vi "Trav_single_profile.vi"(3 "Simulate/Run":T1, 5 "Traverse line":T2 {"Row Duration (mins)" format="%#.1f"; "Row No" min=0; "Trace Gas Concentration (%)" min=0.0 format="%#.2f"; "Emission Rate (l/min)" format="%#.2f"; "Tunnel Speed" format="%#.2f"; "Start X" format="%#.2f"; "Start Y" format="%#.2f"; "Start Z" format="%#.2f"; "End X" format="%#.2f"; "End Y" format="%#.2f"; "End Z" format="%#.2f"; "Averaging time (min)" min=0.0 format="%#.2f"}) -> (0 "Error Messages":string, 1 "Status":T5, 2 "Traverse line Out":T2 {"Row Duration (mins)" format="%#.1f"; "Row No" min=0; "Trace Gas Concentration (%)" min=0.0 format="%#.2f"; "Emission Rate (l/min)" format="%#.2f"; "Tunnel Speed" format="%#.2f"; "Start X" format="%#.2f"; "Start Y" format="%#.2f"; "Start Z" format="%#.2f"; "End X" format="%#.2f"; "End Y" format="%#.2f"; "End Z" format="%#.2f"; "Averaging time (min)" min=0.0 format="%#.2f"})   [LabVIEW 2011]
uses:
  Gen Trav/Multi_Run_Status.ctl
  Gen Trav/Traverse_cluster.ctl
  Gen Trav/Spacing.ctl
  Controls/Multi_run_mode.ctl
  Controls/User_Specific_mode.ctl
  Controls/Save_Data.ctl
  Controls/Setup.ctl
  ADAM Client/Sub VIs/ADAM Controls/Traverse_Level_State.ctl
  Controls/Overhead.ctl
  Globals/Trav_pos_global.vi
  Globals/Meas_global.vi
panel:
  out "Pause message":string
  in  "Pause":bool
  out "Current position":dbl[](array[numeric]) format="%.2f"
  in  "Stop":bool
  in  "Array of Positions":dbl[][](array[numeric]) format="%.2f"
  out "Abcissa copy":string="Y (mm)"
  out "Abcissa":string="Y (mm)"
  in  "ChannelsToPlot":i32[](listbox)=[1]
  out "Started Profile at:":string="16/9/98 12:33"
  out "Currently on point":i32=9
  out "Means":cluster{dbl[], dbl[]}[](graph)
  out "Turbulence%":cluster{dbl[], dbl[]}[](graph)
  # "X           Y            Z"
  # "Start"
  # "End"
  # "X           Y            Z"
  # "Start"
  # "End"
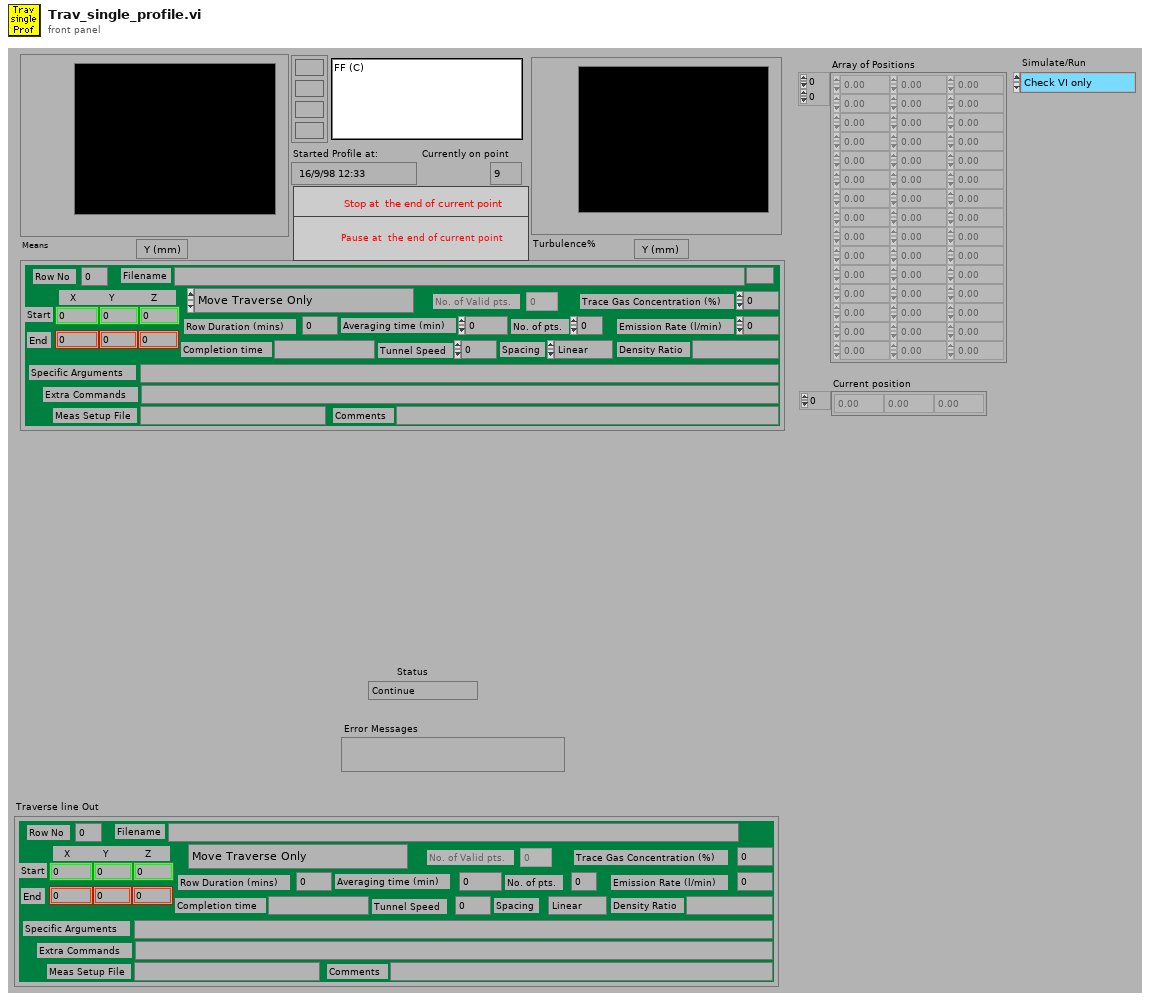
[diagram p1: front panel]
types:
  T1 = typedef "User_Specific_mode.ctl" = enum16{"Check VI only", "Run VI"}
  T2 = typedef "Traverse_cluster.ctl" = cluster{"Start X":dbl, "Start Y":dbl, "Start Z":dbl, "End X":dbl, "End Y":dbl, "End Z":dbl, "No. of pts.":i32, "Spacing":T3, "Filename":path, "Tunnel Speed":dbl, "Averaging time (min)":dbl, "Extra Commands":string, "Specific Arguments":string, "Emission Rate (l/min)":dbl, "Trace Gas Concentration (%)":dbl, "Density Ratio":string, "Comments":string, "Row No":i32, "Row Type Selector":T4, "Completion time":string, "Row Duration (mins)":dbl, "No. of Valid pts.":i32, "Meas Setup File":string}
  T3 = typedef "Spacing.ctl" = enum16{"Linear", "Log", "Gauss", "Specified", "N/A"}
  T4 = typedef "Multi_run_mode.ctl" = enum16{"Move Traverse Only", "Set Tunnel Speed Only", "Set Source Only", "Set Measurement Conditions", "Single Measurement", "Vertical Profile", "Lateral Profile", "Longitudinal Profile", "Explore Volume", "Multi-Axis Profile", "Auto Calibrate", "Meas Fast FID Bkgnd", "Check Beam Power", "Scanning Valve Measurement", "Run VI Named:", "Set ADAM Ch", "Wait (minutes)", "Send Message", "Synchronize With:", "Fall Back to this Row", "Turn Off Row Repeating", "Blank Row", "Traverse 3D Volume"}
  T5 = typedef "Multi_Run_Status.ctl" = enum16{"Continue", "Jump to Next Point", "Jump to Next Row", "Jump To Fall Back", "Terminate Run"}
  T6 = typedef "Save_Data.ctl" = enum16{"Save No Data", "Save Data"}
  T7 = typedef "Setup.ctl" = enum16{"Run Program", "Show Setup", "Save Current Setup", "Setup Front Panel"}
  T8 = typedef "Traverse_Level_State.ctl" = enum16{"Running", "Complete"}
  T9 = typedef "Overhead.ctl" = enum16{"Update total times", "Read Current Overhead", "Re Scale totals to 3 hrs", "Initialise totals to 3hr"}
  T10 = typedef "Status_Cluster.ctl" = cluster{"Status":T5, "Error Type":string, "Error Description":string}
  T11 = typedef "Analysis_info_cluster.ctl" = cluster{"Colour":u32, "Inst type":T12, "Inst name":string, "Symbol":string, "Code name":string, "Extra Info":string, "Inst Array":T13, "Extra Titles":string[], "Extra Values":string[], "Eng Values":dbl[], "Time (ms)":dbl[], "Voltage":dbl[], "U":dbl, "u^2":dbl, "u^3":dbl, "u^4":dbl, "Skew_u":dbl, "Kurt_u":dbl, "Sd Error in Mean":dbl, "% u'/U":dbl, "X":dbl, "Y":dbl, "Z":dbl, "Spectra":T14, "Autocorrelation":T14, "Timescale integral to 25%":dbl, "Sd Error in Variance":dbl, "Calib File":path, "Calib Constants":dbl[], "Histogram":T14, "Output Position":bool, "Full Stats":bool, "Weighting":dbl[], "Av Sampling Rate":dbl, "Av No of Samples":dbl, "Total Meas Time (s)":dbl, "ADAM Ch Name":string}
  T12 = typedef "Inst_type.ctl" = enum16{"Propeller anemometer", "Raw voltage", "Pressure Transducer", "Pitot-static tube", "Preston tube", "Hot wire", "Cross wire 1", "Cross wire 2", "Generic Linear", "Generic Polynomial", "Generic BackPoly", "Fast FID", "Thermocouple", "Cold wire", "Pulsed Wire", "LDA Vel", "LDA Tran time", "LDA Arr time"}
  T13 = typedef "Instrument_Array.ctl" = enum16{"PWA", "LDA", "Analogue"}
  T14 = typedef "XY_Plot_Cluster.ctl" = cluster{"First Name":string, "Second Name":string, "X axis name":string, "Y axis name":string, "X array":dbl[], "Y array":dbl[]}
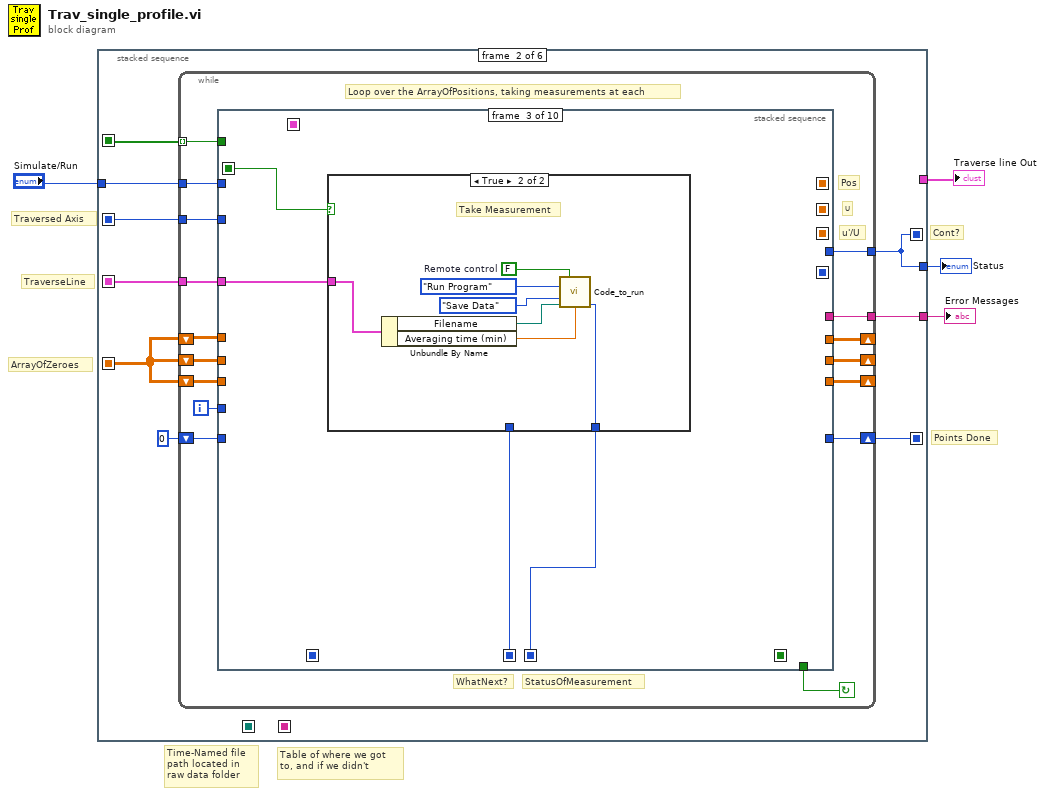
[diagram p0: block diagram]
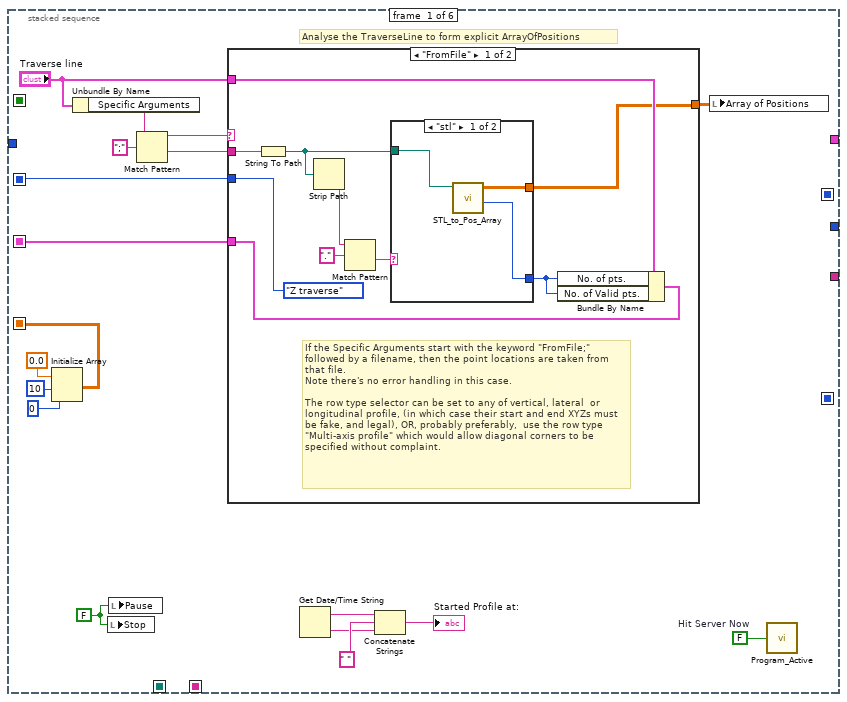
[diagram p2: hidden frame]
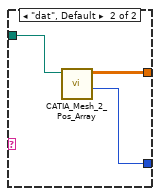
[diagram p3: hidden frame]
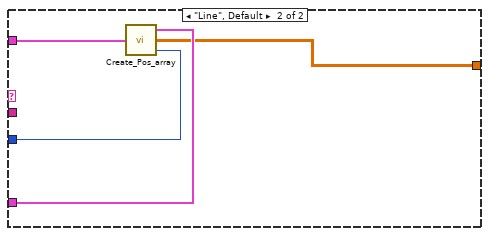
[diagram p4: hidden frame]
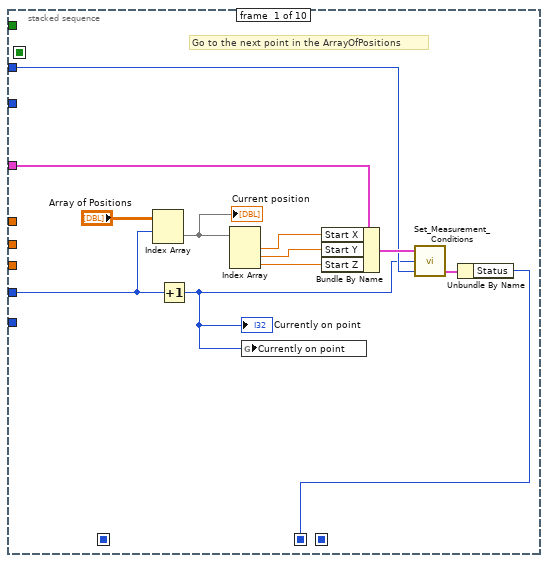
[diagram p5: hidden frame]
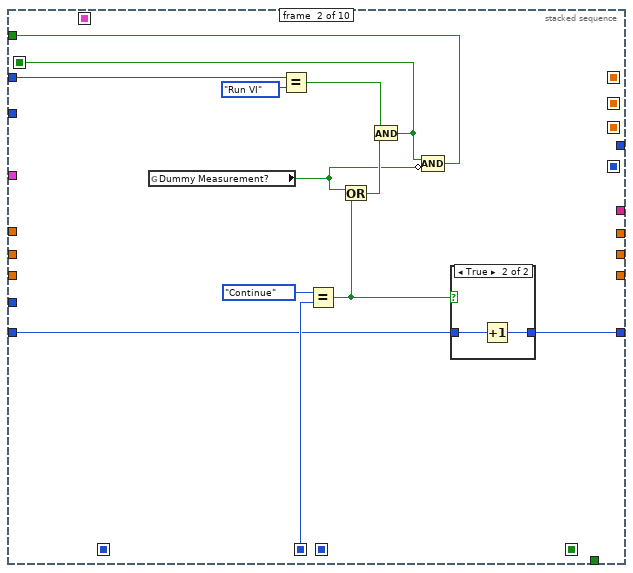
[diagram p6: hidden frame]
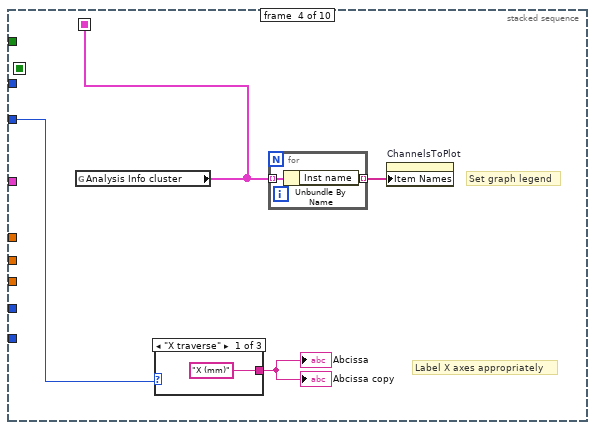
[diagram p9: hidden frame]
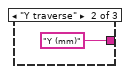
[diagram p10: hidden frame]
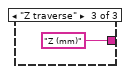
[diagram p11: hidden frame]
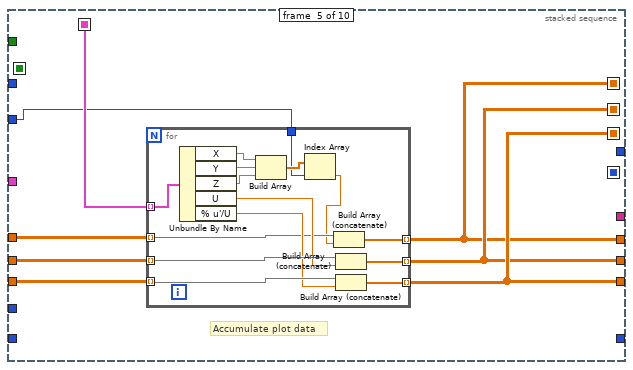
[diagram p12: hidden frame]
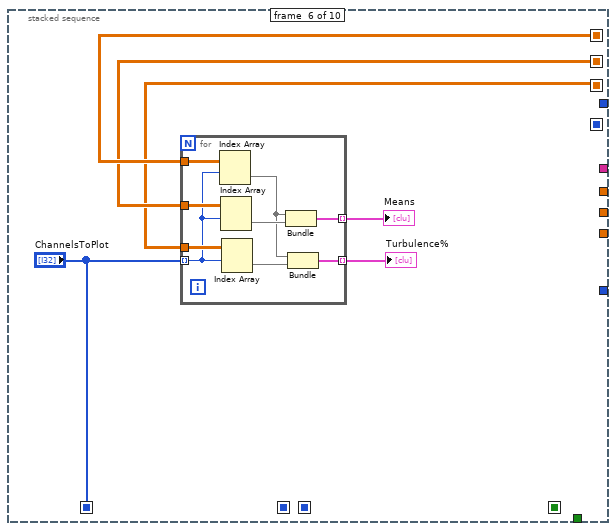
[diagram p13: hidden frame]
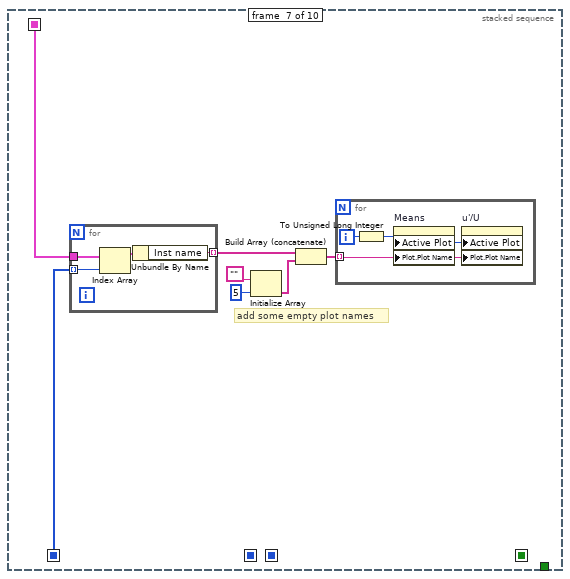
[diagram p14: hidden frame]
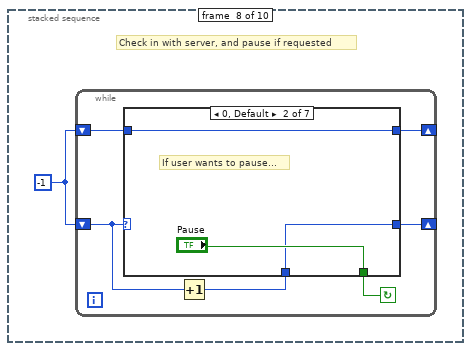
[diagram p15: hidden frame]
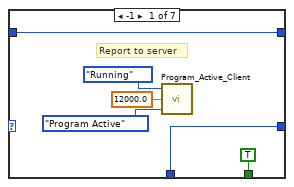
[diagram p16: hidden frame]
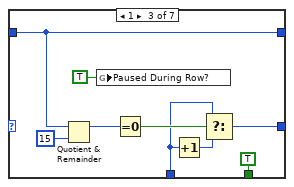
[diagram p17: hidden frame]
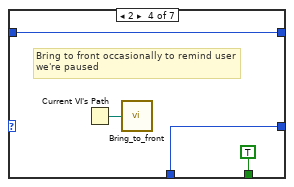
[diagram p18: hidden frame]
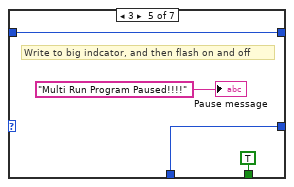
[diagram p19: hidden frame]
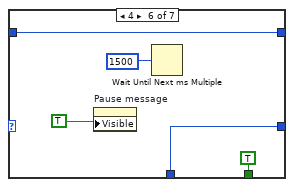
[diagram p20: hidden frame]
diagram:
  # "Table of where we got to, and if we didn't"
  # "Time-Named file path located in raw data folder"
  # "ArrayOfZeroes"
  # "TraverseLine"
  # "Traversed Axis"
  # "Points Done"
  # "Cont?"
  n1 = stacked-sequence {
    seq-local: [w15 _ _ _ _ _] -> [_ w50 _ _ _ _]
    seq-local: [w14 _ _ _ _ _] -> [_ w51 _ _ _ _]
    seq-local: [_ _ w272 _ _ _] -> [_ _ _ _ w296 _]
    seq-local: [_ _ _ w279 _ _] -> [_ _ _ _ w295 _]
    seq-local: [_ w49 _ _ _ _] -> [_ _ _ _ _ _]
    seq-local: [_ w47 _ _ _ _] -> [_ _ _ w276 w294 _]
    seq-local: [_ w45 _ _ _ _] -> [_ _ _ _ _ w301]
    seq-local: [w11 _ _ _ _ _] -> [_ w44 _ _ _ w303]
    tunnel: [_ w49 _ _ _ _] -> w2
    tunnel: [_ _ _ _ _ w313] -> w4
    tunnel: "Simulate/Run" -> [_ w48 _ _ _ w312]
    tunnel: [_ w43 _ _ _ _] -> w1
    frame #0 {
      w12 = FALSE ("stop")
      w13 = FALSE  # Hit Server Now
      # "Analyse the TraverseLine to form explicit ArrayOfPositions"
      n2 = Initialize Array(0.0, 10, 0) -> (w15:dbl[][])
      n3 = Unbundle By Name("Traverse line") -> ("Specific Arguments"=w8:string)
      n4 = local write "Stop"(w12) -> ()
      n5 = local write "Pause"(w12) -> ()
      n6 = Match Pattern(string=w8, regular expression=";") -> (before substring=w6:string, after substring=w5:string)  [unwired: 1 in, 2 out]
      n7 = case shown="\"FromFile\"" w6 {
        tunnel: [enum16{"X traverse", "Y traverse", "Z traverse"}."Z traverse" ("Axis Traversed") w42] -> w14
        tunnel: "Traverse line" -> [w26 w41]
        tunnel: [w25 w40] -> w11
        tunnel: [w23 w39] -> w10
        tunnel: w5 -> [w27 _]
        frame "FromFile" {
          # "If the Specific Arguments start with the keyword \"FromFile;\" followed by a filename, then the point locations are taken from that file.\nNote there's no error handling in this case.\n\nThe row type selector can be set to any of vertical, lateral  or longitudinal profile, (in which case their start and end XYZs must be fake, and legal), OR, probably preferably,  use the row type \"Multi-axis profile\" which would allow diagonal corners to be specified without complaint."
          n8 = String To Path(string=w27) -> (path=w29:path)
          n9 = Strip Path(path=w29) -> (name=w31:string)  [unwired: 1 out]
          n10 = Match Pattern(string=w31, regular expression=".") -> (after substring=w32:string)  [unwired: 1 in, 3 out]
          n11 = case shown="\"stl\"" w32 {
            tunnel: [w34 w38] -> w23
            tunnel: [w33 w37] -> w28
            tunnel: w29 -> [w35 w36]
            frame "stl" {
              n12 = call "STL_to_Pos_Array.vi"("STL file"=w35) -> ("Number of Points"=w33:i32, "Array of Positions"=w34:dbl[][])  [unwired: 9 in]
            }
            frame "dat", Default {
              n13 = call "CATIA_Mesh_2_Pos_Array.vi"("Catia Mesh File"=w36) -> ("Number of Points"=w37:i32, "Array of Positions"=w38:dbl[][])  [unwired: 9 in]
            }
          }
          n14 = Bundle By Name(cluster=w26, "No. of pts."=w28, "No. of Valid pts."=w28) -> (w25:T2)
        }
        frame "Line", Default {
          n15 = call "Create_Pos_array.vi"("Traverse line"=w41) -> ("Traverse line Out"=w40:T2, "Array of Positions"=w39:dbl[][], "Axis Traversed"=w42:enum16{"X traverse", "Y traverse", "Z traverse"})  [unwired: 5 in, 1 out]
        }
      }
      n16 = Get Date/Time String() -> (date string=w21:string, time string=w20:string)  [unwired: 3 out]
      n17 = Concatenate Strings(w21, " ", w20) -> (→"Started Profile at:":string)
      n18 = local write "Array of Positions"(w10) -> ()
      n19 = call "Program_Active.vi"("Hit Server Now"=w13) -> ()
    }
    frame #1 {
      n20 = while {
        shift-left: 0 -> [w54]
        shift-right: [w53] -> w45
        tunnel: [w55] -> w47 mode=indexing
        tunnel: w44 -> [w56]
        tunnel: w48 -> [w57]
        tunnel: [w58] -> w49
        shift-left: w50 -> [w61]
        shift-right: [w60] -> _
        tunnel: w51 -> [w62]
        shift-left: w50 -> [w64]
        shift-right: [w63] -> _
        shift-left: w50 -> [w66]
        shift-right: [w65] -> _
        tunnel: [w52] -> w43
        i -> [w67]
        stop <- w59 continue-if-true
        # "StatusOfMeasurement"
        # "WhatNext?"
        # "Loop over the ArrayOfPositions, taking measurements at each"
        # "Pos"
        # "U"
        # "u'/U"
        n21 = stacked-sequence {
          seq-local: [_ _ _ w107 _ _ _ _ _ _] -> [_ _ _ _ w121 _ w154 _ _ _]
          seq-local: [_ _ _ _ w117 _ _ _ _ _] -> [_ _ _ _ _ w144 _ _ _ _]
          seq-local: [_ _ _ _ w119 _ _ _ _ _] -> [_ _ _ _ _ w143 _ _ _ _]
          seq-local: [_ _ _ _ w120 _ _ _ _ _] -> [_ _ _ _ _ w142 _ _ _ _]
          seq-local: [_ _ _ _ _ "ChannelsToPlot" _ _ _ _] -> [_ _ _ _ _ _ w160 _ _ _]
          seq-local: [_ _ w98 _ _ _ _ _ _ _] -> [_ _ _ _ _ _ _ _ w221 _]
          seq-local: [w74 _ _ _ _ _ _ _ _ _] -> [_ w89 w96 _ _ _ _ _ _ _]
          seq-local: [_ w81 _ _ _ _ _ _ _ _] -> [_ _ w97 _ _ _ _ _ _ _]
          seq-local: [_ _ _ _ _ _ _ _ w216 _] -> [_ _ _ _ _ _ _ _ _ w228]
          seq-local: [_ _ _ _ _ _ _ _ w215 _] -> [_ _ _ _ _ _ _ _ _ w229]
          tunnel: w67 -> [w71 _ _ _ _ _ _ _ w224 w232]
          tunnel: w66 -> [_ _ _ _ w123 _ _ _ _ _]
          tunnel: [_ _ _ _ w119 _ _ _ _ _] -> w65
          tunnel: w64 -> [_ _ _ _ w122 _ _ _ _ _]
          tunnel: [_ _ _ _ w120 _ _ _ _ _] -> w63
          tunnel: w62 -> [_ _ _ w109 w116 _ _ _ _ _]
          tunnel: w61 -> [_ _ _ _ w118 _ _ _ _ _]
          tunnel: [_ _ _ _ w117 _ _ _ _ _] -> w60
          tunnel: [_ _ _ _ _ _ _ _ _ w228] -> w59
          tunnel: w56 -> [w78 _ w95 _ _ _ _ _ _ w233]
          tunnel: [_ _ _ _ _ _ _ _ _ w231] -> w58
          tunnel: w57 -> [w76 w91 _ _ _ _ _ _ _ w234]
          tunnel: [_ w82 _ _ _ _ _ _ _ _] -> w55
          tunnel: w54 -> [_ w86 _ _ _ _ _ _ _ _]
          tunnel: [_ w85 _ _ _ _ _ _ _ _] -> w53
          tunnel: [_ _ _ _ _ _ _ _ _ w230] -> w52
          frame #0 {
            # "Go to the next point in the ArrayOfPositions"
            n22 = Index Array(array="Array of Positions", index (row)=w71) -> (element=w70:dbl[])  [unwired: 1 in]
            "Current position" <- w70
            n23 = Increment(x=w71) -> (x+1=w73:i32)
            "Currently on point" <- w73
            n24 = Index Array(array=w70) -> (element #1=w79:dbl, element #2=w69:dbl, element #3=w68:dbl)  [unwired: 3 in]
            n25 = global write "Trav_pos_global.vi" "Currently on point"(w73) -> ()
            n26 = Bundle By Name(cluster=w78, "Start X"=w79, "Start Y"=w69, "Start Z"=w68) -> (w77:T2)
            n27 = call "Set_Measurement_Conditions.vi"("Simulate/Run"=w76, "Currently on Point"=w73, "Traverse line"=w77) -> ("Status Cluster"=w75:T10)  [unwired: 2 out]
            n28 = Unbundle By Name(w75) -> ("Status"=w74:T5)
          }
          frame #1 {
            n29 = global read "Trav_pos_global.vi" "Dummy Measurement?"() -> (w80:bool)
            n30 = Equal?(x=w91, y=User_Specific_mode."Run VI" ("Simulate/Run")) -> (x = y?=w87:bool)
            n31 = Equal?(x=Multi_Run_Status."Continue" ("Status"), y=w89) -> (x = y?=w84:bool)
            n32 = Or(x=w80, y=w84) -> (x .or. y?=w83:bool)
            n33 = And(x=w87, y=w83) -> (x .and. y?=w81:bool)
            n34 = Compound Arithmetic op=AND(w81, invert w80) -> (w82:bool)
            n35 = case shown="True" w84 {
              tunnel: w86 -> [w92 w94]
              tunnel: [w92 w93] -> w85
              frame False {
              }
              frame True {
                n36 = Increment(x=w94) -> (x+1=w93:i32)
              }
            }
          }
          frame #2 {
            n37 = case shown="True" w97 {
              tunnel: [w99 w106] -> w98
              tunnel: w96 -> [w99 _]
              tunnel: w95 -> [_ w100]
              frame False {
                # "Dummy measurement, or some other reason not to actually measure"
              }
              frame True {
                w105 = FALSE  # Remote control
                # "Take Measurement"
                n38 = Unbundle By Name(w100) -> ("Filename"=w103:path, "Averaging time (min)"=w104:dbl)
                n39 = call "Code_to_run.vi"("setup"=Setup."Run Program", "Remote control"=w105, "File"=Save_Data."Save Data", "Results Filename"=w103, "Averaging time (min)"=w104) -> ("Status"=w106:T5)  [unwired: 6 in, 4 out]
              }
            }
          }
          frame #3 {
            # "Label X axes appropriately"
            # "Set graph legend"
            n40 = global read "Meas_global.vi" "Analysis Info cluster"() -> (w107:T11[])
            n41 = case shown="\"X traverse\"" w109 {
              tunnel: ["X (mm)" "Y (mm)" "Z (mm)"] -> w108
              frame "X traverse" {
              }
              frame "Y traverse" {
              }
              frame "Z traverse" {
              }
            }
            "Abcissa" <- w108
            "Abcissa copy" <- w108
            n42 = for {
              tunnel: w107 -> [w115] mode=indexing
              tunnel: [w114] -> w110 mode=indexing
              n43 = Unbundle By Name(w115) -> ("Inst name"=w114:string)
            }
            n44 = property on="ChannelsToPlot" class="LstBox (strict)"("Item Names"=w110) -> ()  [unwired: 2 in, 2 out]
          }
          frame #4 {
            # "Accumulate plot data"
            n45 = for {
              tunnel: w123 -> [w138] mode=indexing
              tunnel: [w136] -> w119 mode=indexing
              tunnel: w122 -> [w135] mode=indexing
              tunnel: [w133] -> w120 mode=indexing
              tunnel: w121 -> [w132] mode=indexing
              tunnel: w118 -> [w131] mode=indexing
              tunnel: [w130] -> w117 mode=indexing
              tunnel: w116 -> [w125]
              n46 = Unbundle By Name(w132) -> ("X"=w129:dbl, "Y"=w128:dbl, "Z"=w127:dbl, "U"=w137:dbl, "% u'/U"=w134:dbl)
              n47 = Build Array(w129, w128, w127) -> (w126:dbl[])
              n48 = Index Array(array=w126, index=w125) -> (element=w124:dbl)
              n49 = Build Array (concatenate)(w131, w124) -> (w130:dbl[])
              n50 = Build Array (concatenate)(w138, w137) -> (w136:dbl[])
              n51 = Build Array (concatenate)(w135, w134) -> (w133:dbl[])
            }
          }
          frame #5 {
            n52 = for {
              tunnel: "ChannelsToPlot" -> [w145] mode=indexing
              tunnel: w144 -> [w153]
              tunnel: w143 -> [w152]
              tunnel: w142 -> [w151]
              tunnel: [w147] -> w141 mode=indexing
              tunnel: [w146] -> w140 mode=indexing
              n53 = Index Array(array=w153, index (row)=w145) -> (element=w149:dbl[])  [unwired: 1 in]
              n54 = Index Array(array=w152, index (row)=w145) -> (element=w150:dbl[])  [unwired: 1 in]
              n55 = Index Array(array=w151, index (row)=w145) -> (element=w148:dbl[])  [unwired: 1 in]
              n56 = Bundle(w149, w150) -> (w146:cluster{dbl[], dbl[]})  [unwired: 1 out]
              n57 = Bundle(w149, w148) -> (w147:cluster{dbl[], dbl[]})  [unwired: 1 out]
            }
            "Means" <- w140
            "Turbulence%" <- w141
          }
          frame #6 {
            # "add some empty plot names"
            n58 = for {
              tunnel: w160 -> [w164] mode=indexing
              tunnel: w154 -> [w162]
              tunnel: [w161] -> w157 mode=indexing
              n59 = Index Array(array=w162, index=w164) -> (element=w163:T11)
              n60 = Unbundle By Name(w163) -> ("Inst name"=w161:string)
            }
            n61 = Initialize Array("", 5) -> (w156:string[])
            n62 = Build Array (concatenate)(w157, w156) -> (w155:string[])
            n63 = for {
              tunnel: w155 -> [w165] mode=indexing
              i -> [w167]
              n64 = To Unsigned Long Integer(number=w167) -> (unsigned 32bit integer=w166:u32)
              n65 = property on="Means" class="XYGraph (strict)"("Active Plot"=w166, "Plot.Plot Name"=w165) -> ()  [unwired: 2 in, 2 out]
              n66 = property on="u'/U" class="XYGraph (strict)"("Active Plot"=w166, "Plot.Plot Name"=w165) -> ()  [unwired: 2 in, 2 out]
            }
          }
          frame #7 {
            w168 = -1
            # "Check in with server, and pause if requested"
            n67 = while {
              shift-left: w168 -> [w169]
              shift-right: [w170] -> _
              shift-left: w168 -> [w173]
              shift-right: [w174] -> _
              stop <- w171 continue-if-true
              n68 = Increment(x=w173) -> (x+1=w172:i32)
              n69 = case shown="0, Default" w173 {
                tunnel: [w179 w182 w186 w196 w199 w203 0] -> w174
                tunnel: w172 -> [w179 w182 w188 w196 w199 w203 _]
                tunnel: [TRUE ("Pause") "Pause" TRUE ("Pause") TRUE ("Pause") TRUE ("Pause") TRUE ("Pause") TRUE ("Pause")] -> w171
                tunnel: [w178 w181 w184 w193 w197 w201 w206] -> w170
                tunnel: w169 -> [w178 w181 w184 w193 w197 w201 w207]
                frame -1 {
                  # "Report to server"
                  n70 = call "Program_Active_Client.vi"("Mode"=enum16{"Program Active", "Traverse Level State"}."Program Active", "Time till next contact (Sec)"=12000.0, "Traverse level State"=Traverse_Level_State."Running") -> ()  [unwired: 3 out]
                }
                frame 0, Default {
                  # "If user wants to pause..."
                }
                frame 1 {
                  n71 = Quotient & Remainder(x=w184, y=15) -> (x-y*floor(x/y)=w190:i32)  [unwired: 1 out]
                  n72 = global write "Trav_pos_global.vi" "Paused During Row?"(TRUE ("Paused During Row?")) -> ()
                  n73 = Equal To 0?(x=w190) -> (x = 0?=w189:bool)
                  n74 = Increment(x=w188) -> (x+1=w187:i32)
                  n75 = Select(t=w188, s=w189, f=w187) -> (s? t:f=w186:i32)
                }
                frame 2 {
                  # "Bring to front occasionally to remind user we're paused"
                  n76 = Current VI's Path() -> (path=w194:path)
                  n77 = call "Bring_to_front.vi"("path"=w194) -> ()
                }
                frame 3 {
                  # "Write to big indcator, and then flash on and off"
                  "Pause message" <- "Multi Run Program Paused!!!!" ("Pause message")
                }
                frame 4 {
                  n78 = property on="Pause message" class="Str"("Visible"=TRUE) -> ()  [unwired: 2 in, 2 out]
                  n79 = Wait Until Next ms Multiple(millisecond multiple=u32 1500) -> ()  [unwired: 1 out]
                }
                frame 5 {
                  n80 = Increment(x=w207) -> (x+1=w206:i32)
                  n81 = property on="Pause message" class="Str"("Visible"=FALSE) -> ()  [unwired: 2 in, 2 out]
                  n82 = Wait Until Next ms Multiple(millisecond multiple=u32 1500) -> ()  [unwired: 1 out]
                }
              }
            }
          }
          frame #8 {
            n83 = local read "Array of Positions"() -> (w217:dbl[][])
            n84 = Array Size(array=w217) -> (size(s)=w220:i32[])
            n85 = Index Array(array=w220, index=0 ("Index")) -> (element=w218:i32)
            n86 = Increment(x=w224) -> (x+1=w223:i32)
            n87 = Less?(x=w223, y=w218) -> (x < y?=w213:bool)
            n88 = case shown="\"Jump to Next Point\"" w221 {
              tunnel: [TRUE TRUE FALSE] -> w212
              frame "Continue" {
              }
              frame "Jump to Next Point" {
              }
              frame "Jump to Next Row", Default {
              }
            }
            n89 = Compound Arithmetic op=AND(invert "Stop", w213, w212) -> (w216:bool)
            n90 = Select(t=Multi_Run_Status."Terminate Run" ("Status"), s="Stop", f=w221) -> (s? t:f=w215:T5)
          }
          frame #9 {
            n91 = case shown="True" w228 {
              tunnel: w234 -> [_ w243]
              tunnel: w233 -> [_ w242]
              tunnel: w232 -> [_ w241]
              tunnel: [w236 w238] -> w231
              tunnel: ["" w237] -> w230
              tunnel: w229 -> [w236 _]
              frame False {
                # "No more points to do...."
              }
              frame True {
                n92 = case shown="\"Check VI only\"" w243 {
                  tunnel: w242 -> [w259 _]
                  tunnel: w241 -> [w254 _]
                  tunnel: [w246 timestamp(0 s since 1904-01-01)] -> w240
                  frame "Check VI only" {
                    n93 = Unbundle By Name(w259) -> ("Averaging time (min)"=w256:dbl)
                    n94 = global read "Trav_pos_global.vi" "Simulation Time"() -> (w248:timestamp)
                    n95 = Multiply(x=60.0, y=w256) -> (x*y=w255:dbl)
                    n96 = To Double Precision Float(number=w248) -> (double precision float=w249:dbl)
                    n97 = Add(x=w255, y=10.0 ("Scalable Time (Sec)")) -> (x+y=w253:dbl)
                    n98 = Increment(x=w254) -> (x+1=w252:i32)
                    n99 = call "Overhead_Factor.vi"("Mode"=Overhead."Read Current Overhead") -> ("Current Overhead Factor"=w244:dbl)  [unwired: 3 in]
                    n100 = Multiply(x=w253, y=w252) -> (x*y=w245:dbl)
                    n101 = Multiply(x=w245, y=w244) -> (x*y=w250:dbl)
                    n102 = Add(x=w249, y=w250) -> (x+y=w247:dbl)
                    n103 = To Time Stamp(1:w247) -> (0:w246:timestamp)
                  }
                  frame "Run VI" {
                  }
                }
                n104 = call "Run_FFID_Bkgnd.vi"("Simulated Time"=w240, "Run Now?"=FALSE, "Simulate/Run"=w243) -> ("Error Messages"=w237:string, "Status"=w238:T5)  [unwired: 1 out]
              }
            }
          }
        }
      }
    }
    frame #2 {
      n105 = global read "Meas_global.vi" "Start Time of experiment"() -> (w262:dbl)
      n106 = global read "Meas_global.vi" "Raw data file"() -> (w274:path)
      n107 = Strip Path(path=w274) -> (stripped path=w273:path)  [unwired: 1 out]
      n108 = call "Sec_to_date_filename.vi"("seconds"=w262) -> ("Day"=w264:string, "Time"=w265:string)  [unwired: 2 out]
      n109 = Format Into String(format string="Cmd_%s_%s.xls", w264, w265) -> (resulting string=w267:string)  [unwired: 2 in, 1 out]
      n110 = call "Fast_string_Replace.vi"("Replace match with:"="-", "Input String"=w267, "regular expression"=":") -> ("Output String"=w270:string)  [unwired: 2 out]
      n111 = call "Fast_string_Replace.vi"("Replace match with:"="", "Input String"=w270, "regular expression"=" ") -> ("Output String"=w261:string)  [unwired: 2 out]
      n112 = Build Path(base path=w273, name or relative path=w261) -> (appended path=w272:path)
    }
    frame #3 {
      w285 = "\t"
      n113 = local read "Array of Positions"() -> (w278:dbl[][])
      n114 = Number To Fractional String(number=w278, precision (6)=i16 2) -> (F-format string=w277:string[][])  [unwired: 2 out]
      n115 = for {
        tunnel: w277 -> [w290] mode=indexing
        tunnel: w276 -> [w289] mode=indexing
        tunnel: [w287] -> w275 mode=indexing
        n116 = case shown="True" w289 {
          tunnel: ["Unobtainable Position" ""] -> w288
          frame False {
          }
          frame True {
          }
        }
        n117 = Build Array (concatenate)(w290, w288) -> (w287:string[])
      }
      n118 = Concatenate Strings("X", w285, "Y", w285, "Z") -> (w280:string)
      n119 = call "2D_array_to_string.vi"("2D data array"=w275, "Column titles  (separated by tabs)"=w280, "Array title"="Requested positions") -> ("Output string"=w279:string)
    }
    frame #4 {
      n120 = Or Array Elements(Boolean array=w294) -> (logical OR=w293:bool)
      n121 = case shown="True" w293 {
        tunnel: w296 -> [_ w299]
        tunnel: w295 -> [_ w297]
        frame False {
        }
        frame True {
          w298 = FALSE  # Lock File
          w300 = TRUE  # append to file? (new file:F)
          # "If we managed to get to even one point, write a file"
          n122 = call "Write_Characters_To_File.vi"("file path (dialog if empty)"=w299, "character string"=w297, "append to file? (new file:F)"=w300, "Lock File"=w298) -> ()  [unwired: 1 in, 4 out]
        }
      }
    }
    frame #5 {
      n123 = local read "Array of Positions"() -> (w305:dbl[][])
      n124 = Array Size(array=w305) -> (size(s)=w307:i32[])
      n125 = Index Array(array=w307, index=0 ("Index")) -> (element=w304:i32)
      n126 = Not Equal?(x=w304, y=w301) -> (x != y?=w310:bool)
      n127 = Equal?(x=User_Specific_mode."Run VI" ("Simulate/Run"), y=w312) -> (x = y?=w309:bool)
      n128 = Bundle By Name(cluster=w303, "No. of Valid pts."=w301) -> (w302:T2)
      n129 = And(x=w309, y=w310) -> (x .and. y?=w308:bool)
      n130 = case shown="True" w308 {
        tunnel: w302 -> [w314 w326]
        tunnel: [w314 w325] -> w313
        tunnel: w301 -> [_ w324]
        frame False {
        }
        frame True {
          w315 = " !!Program added comments"
          n131 = Unbundle By Name(w326) -> ("Comments"=w316:string)
          n132 = Equal To 0?(x=w324) -> (x = 0?=w323:bool)
          n133 = Select(t=" !!(Row Skipped)", s=w323, f=" !!(Row Partially Skipped)") -> (s? t:f=w319:string)
          n134 = Match Pattern(string=w316, regular expression=w315) -> (match substring=w318:string)  [unwired: 4 out]
          n135 = Empty String/Path?(string/path=w318) -> (empty?=w317:bool)
          n136 = case shown="False" w317 {
            tunnel: [w329 w333] -> w320
            tunnel: w319 -> [w328 w332]
            tunnel: w315 -> [_ w331]
            tunnel: w316 -> [w327 w330]
            frame False {
              n137 = Concatenate Strings(w327, w328) -> (w329:string)
            }
            frame True {
              n138 = Concatenate Strings(w330, w331, w332) -> (w333:string)
            }
          }
          n139 = Bundle By Name(cluster=w326, "Comments"=w320) -> (w325:T2)
        }
      }
    }
  }
  "Status" <- w2
  "Traverse line Out" <- w4
  "Error Messages" <- w1
